vi "Simulacion_FOPID_Aproximados.vi"() -> ()   [LabVIEW 2019]
uses:
  <vilib>/Simulation/Scripting/Companion Diagram/SimConfigNode/SimParams.ctl
  <vilib>/Simulation/Scripting/Companion Diagram/SimConfigNode/_simSolvers.ctl
  <vilib>/Simulation/Implementation/Shared/SIMSCR Execution Mode.ctl
  <vilib>/Simulation/Param Hierarchy/Typedefs/SIMPH Param Control Actions.ctl
  <vilib>/Simulation/Implementation/Shared/NILVSim_ParamChanged.vi
  <vilib>/Simulation/Implementation/Shared/NILVSIM_BeginStep.vi
  <vilib>/Simulation/DataSources/Implementation/NILVSim Step.llb/SIM Step (scalar).vi
  <vilib>/Simulation/ContinuousLinear/Implementation/NILVSim Transfer Function.llb/SIM Transfer Function Distributor (SISO CD).vi
  <vilib>/Simulation/SignalArithmetic/Implementation/NILVSim Gain.llb/SIM Gain (scalar).vi
  <vilib>/Simulation/Implementation/Shared/SIM Is Init or Final Stage.vi
  <vilib>/Simulation/ContinuousLinear/Implementation/NILVSim Transfer Function Direct.llb/SIM Transfer Function Direct (SISO).vi
  <vilib>/Simulation/DiscreteLinear/Implementation/NILVSim Discrete Transfer Function Direct.llb/SIM Discrete Transfer Function Direct (SISO).vi
  <vilib>/Simulation/ContinuousLinear/Implementation/NILVSim Transfer Function.llb/SIM Transfer Function Collector (SISO).vi
  <vilib>/Simulation/Implementation/Shared/NILVSim_Manager.vi
  <vilib>/Utility/error.llb/Clear Errors.vi
  <vilib>/Simulation/Implementation/Shared/NILVSim_FinalizeModel.vi
  <vilib>/Simulation/Implementation/Shared/SIM Unbundle Sim Info.vi
  <vilib>/Simulation/Implementation/Shared/NILVSim_Initialize.vi
  <vilib>/addons/Control Design/_Model Construction/Model Creation.llb/CD Construct Transfer Function Model.vi
  <vilib>/addons/Control Design/_Model Construction/Model Creation.llb/Model Creation SubVI/cd_Create Symbolic Transfer Function Model.vi
  <vilib>/Simulation/Utility/Implementation/NILVSim Get Time and IsAcceptedStep.vi
  <vilib>/Simulation/Implementation/Shared/SIMSH Read Queue.vi
  <vilib>/Simulation/Implementation/Shared/NILVSim_GetModelError.vi
  <vilib>/Simulation/Implementation/Shared/SIM Bundle Sim Info.vi
  <vilib>/Simulation/Scripting/Companion Diagram/SimConfigNode/SimDog.xnode
  <vilib>/Simulation/Implementation/XNodeFramework/SimXNode/SimX.xnode
  <vilib>/addons/Control Design/_Model Construction/Model Typedefs.llb/CD Transfer Function Model (SISO).ctl
  <vilib>/addons/Control Design/_Model Construction/NI_LinSys_Model Typedefs.lvlib
  <vilib>/addons/Control Design/_Model Construction/Model Typedefs.llb/CD General Elements.ctl
  <vilib>/addons/Control Design/_Model Construction/Model Typedefs.llb/CD Transfer Function Model (MIMO).ctl
  <vilib>/addons/Control Design/_Model Construction/NI_LinSys_Model Creation.lvlib
  <vilib>/Simulation/ContinuousLinear/Implementation/NILVSim Transfer Function.llb/SIM Transfer Function (SISO CD).vi
  <vilib>/Simulation/Implementation/Shared/NI_SIM_Implementation.lvlib
panel:
  in  "Controlador FOPID":T1(ring)
  in  "L":string="0.0002798"
  in  "T":dbl=0.0045916
  in  "K":dbl=7586.4
  out "Respuesta temporal del Sistema de Control FOPID":cluster{"output":dbl, "output y(t)":dbl}(graph)={"output"=0.0, "output y(t)"=0.6204389612912122}
  out "Velocidad \n(rpm)":dbl=0.6204389612912122
  in  "Set Point (rpm)":dbl(slide) scale=0.0..3500.0
  # "MEJORES CONTROLADORES FOPID"
  # "Parámetros de la Planta (Motor DC)"
  # "DESCRIPCIÓN\nVP: Variable del proceso.\nSP: Set Point / VAlor deseado.\n- Parámetros de la planta: Parametros de un modelo de primer con tiempo de retardo. (motor dc).\n- Controlador FOPID: Se selecciona el controlador FOPID para simular el sistema de control.\n- Respuesta temporal del sistema de control FOPID: visualiza la grafica de la respuesta del sistema\n   de control.\n- Para simular el sistema de control variar el valor de la variable Set Point o en su defecto el slider y     \n   seleccionar el controlador FOPID que se desea simular."
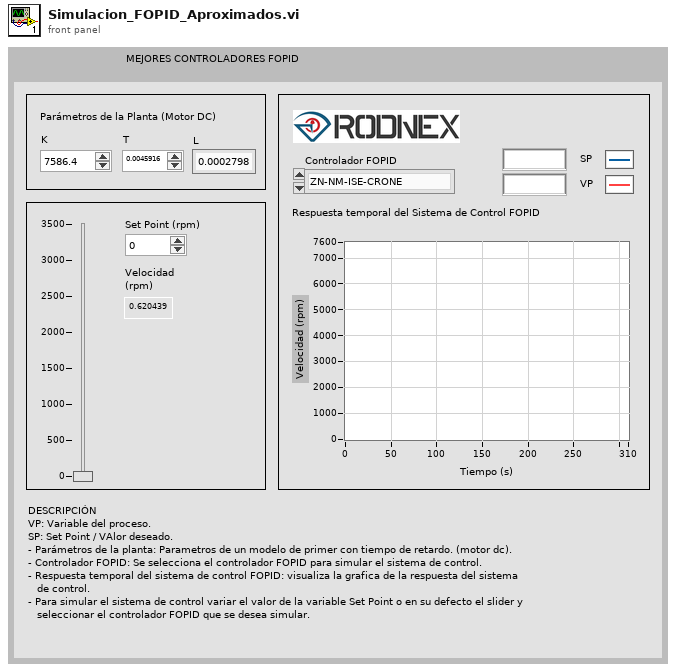
[diagram p1: front panel]
types:
  T1 = enum16{"ZN-NM-ISE-CRONE", "ZN-NM-IAE-CRONE", "ZN-NM-ITSE-CRONE", "ZN-IP-IAE-CARLSON", "ZN-IP-IAE-MATSUDA", "ZN-IP-ISE-MATSUDA", "ZN-IP-ITSE-CARLSON", "ZN-SQP-ISE-MATSUDA", "ZN-SQP-IAE-MATSUDA", "ZN-SQP-ITSE-MATSUDA", "ZN-SQP-ITAE-MATSUDA"}
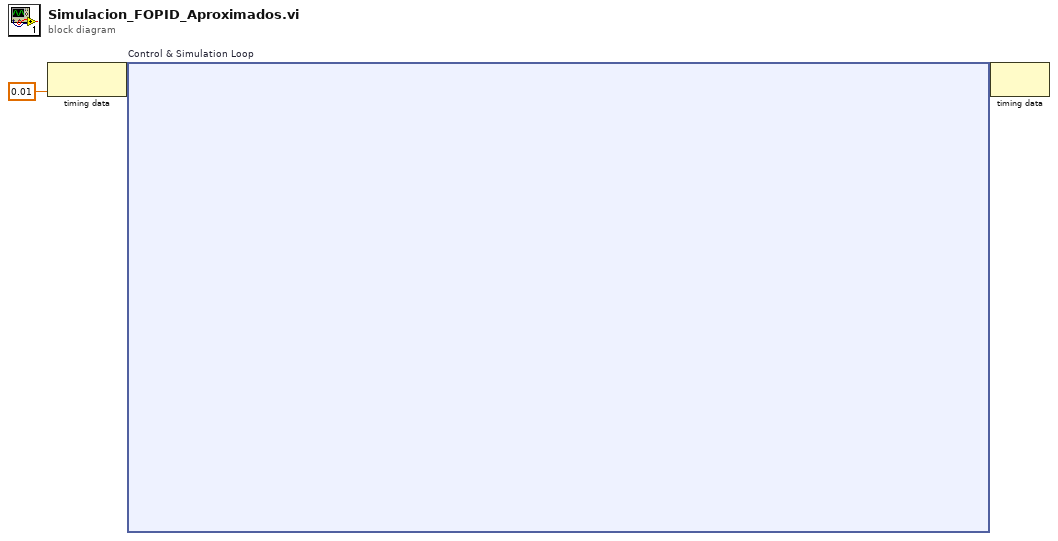
[diagram p0: block diagram]
diagram:
  n1 = node-c288(0.01 ("Discrete Step Size (s)")) -> (w3:variant)
  n2 = node-c254 "Control & Simulation Loop"(w3) -> (w2:variant)
  n3 = node-c288(w2) -> ()  [unwired: 1 out]
